vi "DT_Merge_Main.vi"(5 "left/right pt (right:F)":bool, 9 "Data In":T1, 10 "Triangles In":i32[][](array[numeric]), 11 "Points In":cluster{"x":dbl, "y":dbl, "index":i32}[](array[cluster])) -> (0 "triangle":i32, 1 "Data Out":T1, 2 "Triangles Out":i32[][](array[numeric]), 3 "Points Out":cluster{"x":dbl, "y":dbl, "index":i32}[](array[cluster]), 4 "point":i32)   [LabVIEW 2017, in "NI_AAL_Geometry.lvlib"]
uses:
  <vilib>/Analysis/NI_AAL_Geometry.lvlib
  <vilib>/Analysis/geometry.llb/DT_Merge_Find Next Triangulation_Data.ctl
  <vilib>/Analysis/geometry.llb/DT_Cal Length.vi
  <vilib>/Analysis/baseanly.llb/Determinant.vi
  <vilib>/Analysis/baseanly.llb/Real Determinant.vi
  <vilib>/Analysis/geometry.llb/DT_Triangle Manager_Get Adj_by Point.vi
  <vilib>/Analysis/geometry.llb/DT_Triangle Manager_Get Adj Ghost.vi
  <vilib>/Analysis/geometry.llb/DT_Triangle Manager_Get Adj Point_by Edge.vi
  <vilib>/Analysis/geometry.llb/DT_Triangle Manager_Format Ghost.vi
  <vilib>/Analysis/geometry.llb/DT_Triangle Manager_Get Oppo Point_in Ghost.vi
  <vilib>/Analysis/geometry.llb/DT_Triangle Manager_Get Oppo Point.vi
  <vilib>/Analysis/geometry.llb/DT_Triangle Manager_Default Ghost Index.vi
  <vilib>/Analysis/geometry.llb/DT_Triangle Manager_Get Ghost Point.vi
  <vilib>/Analysis/geometry.llb/DT_Triangle Manager_Get Oppo Edge.vi
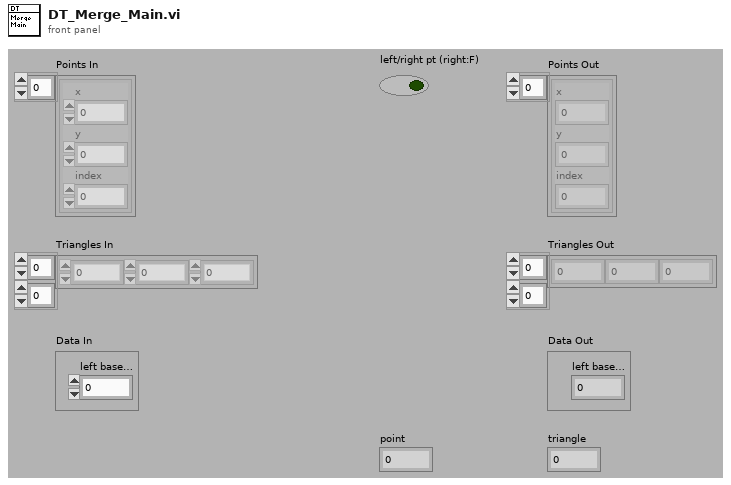
[diagram p1: front panel]
types:
  T1 = typedef "NI_AAL_Geometry.lvlib/DT_Merge_Find Next Triangulation_Data.ctl" = cluster{"left base point":i32, "left triangle":i32, "left local idx":i32, "right base point":i32, "right triangle":i32, "right local idx":i32, "Left Candidate Triangles":i32[], "Left Candidate Point Idx":i32[], "Right Candidate Triangles":i32[], "Right Candidate Point Idx":i32[], "cur triangle":i32}
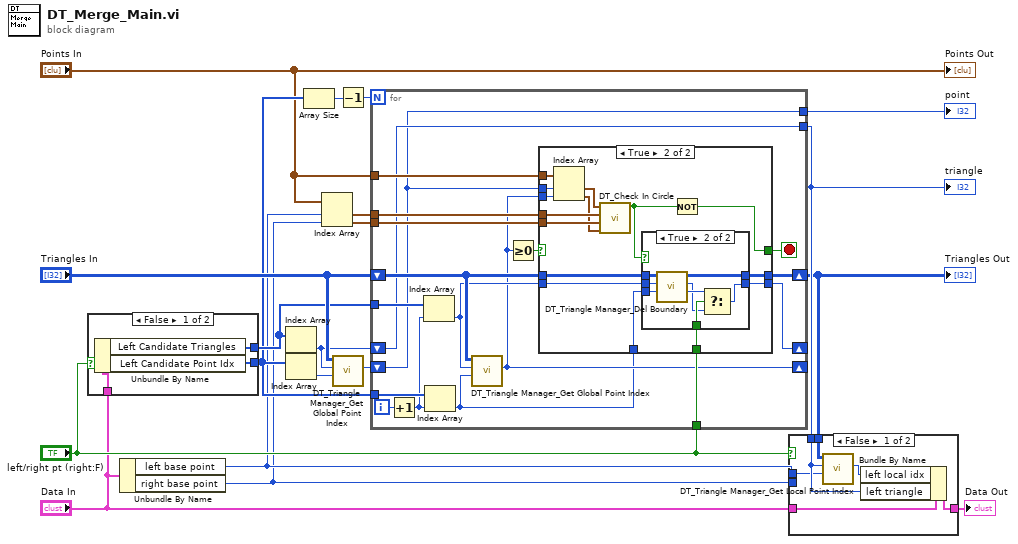
[diagram p0: block diagram]
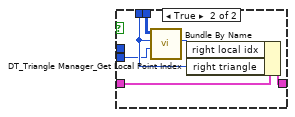
[diagram p2: hidden frame]
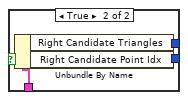
[diagram p3: hidden frame]
diagram:
  n1 = case shown="False" "left/right pt (right:F)" {
    tunnel: [w22 w25] -> w11
    tunnel: "Data In" -> [w21 w24]
    tunnel: [w20 w23] -> w12
    frame False {
      n2 = Unbundle By Name(w21) -> ("Left Candidate Triangles"=w20:i32[], "Left Candidate Point Idx"=w22:i32[])
    }
    frame True {
      n3 = Unbundle By Name(w24) -> ("Right Candidate Triangles"=w23:i32[], "Right Candidate Point Idx"=w25:i32[])
    }
  }
  n4 = Unbundle By Name("Data In") -> ("left base point"=w4:i32, "right base point"=w3:i32)
  n5 = Index Array(array=w12) -> (element=w13:i32)  [unwired: 1 in]
  n6 = Index Array(array=w11) -> (element=w14:i32)  [unwired: 1 in]
  n7 = Array Size(array=w11) -> (size(s)=w19:i32)
  n8 = Index Array(array="Points In", index #1=w4, index #2=w3) -> (element #1=w18:cluster{"x":dbl, "y":dbl, "index":i32}, element #2=w17:cluster{"x":dbl, "y":dbl, "index":i32})
  n9 = call <vilib>:"DT_Triangle Manager_Get Global Point Index.vi"("local idx"=w14, "triangle"=w13, "Triangles"="Triangles In") -> ("global idx"=w5:i32)  [unwired: 8 out]
  n10 = Decrement(x=w19) -> (x-1=w15:i32)
  n11 = for {
    N: w15 -> [_]
    tunnel: w11 -> [w42]
    tunnel: w18 -> [w40]
    tunnel: w17 -> [w39]
    shift-right: [w38] -> w6
    shift-left: "Triangles In" -> [w35]
    tunnel: w12 -> [w36]
    shift-right: [w27] -> _
    shift-left: w5 -> [w31]
    tunnel: [w32] -> w7
    tunnel: [w31] -> w2
    shift-right: [w29] -> _
    shift-left: w13 -> [w32]
    tunnel: "left/right pt (right:F)" -> [w28]
    tunnel: "Points In" -> [w41]
    i -> [w43]
    stop <- w33 stop-if-true
    n12 = Increment(x=w43) -> (x+1=w37:i32)
    n13 = Index Array(array=w36, index=w37) -> (element=w30:i32)
    n14 = Index Array(array=w42, index=w37) -> (element=w26:i32)
    n15 = call <vilib>:"DT_Triangle Manager_Get Global Point Index.vi"("local idx"=w26, "triangle"=w30, "Triangles"=w35) -> ("global idx"=w27:i32)  [unwired: 8 out]
    n16 = Greater Or Equal To 0?(x=w27) -> (x >= 0?=w34:bool)
    n17 = case shown="True" w34 {
      selector: w34 -> [w46 _]
      tunnel: w41 -> [_ w61]
      tunnel: w40 -> [_ w59]
      tunnel: w39 -> [_ w58]
      tunnel: [w45 w56] -> w38
      tunnel: w27 -> [_ w55]
      tunnel: w31 -> [_ w54]
      tunnel: w35 -> [w45 w53]
      tunnel: w30 -> [w44 w50]
      tunnel: [w46 w51] -> w33
      tunnel: [w44 w49] -> w29
      tunnel: w28 -> [_ w48]
      tunnel: w26 -> [_ w47]
      frame False {
      }
      frame True {
        n18 = Index Array(array=w61, index #1=w54, index #2=w55) -> (element #1=w60:cluster{"x":dbl, "y":dbl, "index":i32}, element #2=w57:cluster{"x":dbl, "y":dbl, "index":i32})
        n19 = call <vilib>:"DT_Check In Circle.vi"("p 4"=w57, "p 3"=w58, "p 2"=w59, "p 1"=w60) -> ("in circle?"=w52:bool)  [unwired: 7 out]
        n20 = case shown="True" w52 {
          tunnel: w53 -> [w63 w71]
          tunnel: [w63 w70] -> w56
          tunnel: w50 -> [w62 w69]
          tunnel: w47 -> [_ w68]
          tunnel: [w62 w64] -> w49
          tunnel: w48 -> [_ w67]
          frame False {
          }
          frame True {
            n21 = call <vilib>:"DT_Triangle Manager_Del Boundary.vi"("point idx"=w68, "triangle in"=w69, "Triangles In"=w71) -> ("adj triangle"=w66:i32, "triangle out"=w65:i32, "Triangles Out"=w70:i32[][])  [unwired: 6 out]
            n22 = Select(t=w66, s=w67, f=w65) -> (s? t:f=w64:i32)
          }
        }
        n23 = Not(x=w52) -> (.not. x?=w51:bool)
      }
    }
  }
  "Triangles Out" <- w6
  "triangle" <- w7
  "point" <- w2
  n24 = case shown="False" "left/right pt (right:F)" {
    tunnel: "Data In" -> [w77 w83]
    tunnel: [w76 w82] -> w8
    tunnel: w7 -> [w74 w80]
    tunnel: w6 -> [w75 w81]
    tunnel: w4 -> [w73 _]
    tunnel: w3 -> [_ w78]
    frame False {
      n25 = call <vilib>:"DT_Triangle Manager_Get Local Point Index.vi"("global idx"=w73, "triangle"=w74, "Triangles"=w75) -> ("local idx"=w72:i32)  [unwired: 8 out]
      n26 = Bundle By Name(cluster=w77, "left local idx"=w72, "left triangle"=w74) -> (w76:T1)
    }
    frame True {
      n27 = call <vilib>:"DT_Triangle Manager_Get Local Point Index.vi"("global idx"=w78, "triangle"=w80, "Triangles"=w81) -> ("local idx"=w79:i32)  [unwired: 8 out]
      n28 = Bundle By Name(cluster=w83, "right local idx"=w79, "right triangle"=w80) -> (w82:T1)
    }
  }
  "Data Out" <- w8
  "Points Out" <- "Points In"
